vi "prac2-2.vi"() -> ()   [LabVIEW 2014]
panel:
  out "y":dbl
  out "x":dbl
  in  "stop":bool
  out "XY Graph":cluster{dbl[], dbl[]}(graph)
  in  "L2":dbl
  in  "L1":dbl
  in  "Angulo 2":dbl(knob)
  in  "Angulo 1":dbl(knob)
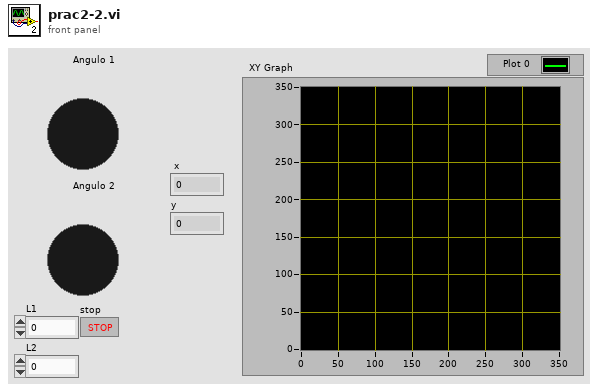
[diagram p1: front panel]
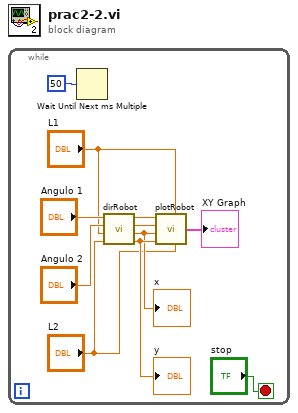
[diagram p0: block diagram]
diagram:
  n1 = while {
    stop <- "stop" stop-if-true
    n2 = Wait Until Next ms Multiple(millisecond multiple=u32 50) -> ()  [unwired: 1 out]
    n3 = call "dirRobot.vi"("L2"="L2", "L1"="L1", "Angulo 2"="Angulo 2", "Angulo 1"="Angulo 1") -> ("y"=w11:dbl, "x"=w10:dbl, "y1"=w9:dbl, "x1"=w8:dbl)
    "x" <- w10
    "y" <- w11
    n4 = call "plotRobot.vi"("L2"="L2", "L1"="L1", "y"=w11, "x"=w10, "y1"=w9, "x1"=w8) -> ("XY Graph"=→"XY Graph":cluster{dbl[], dbl[]})  [unwired: 2 in]
  }
